vi "Create Channel.vi"(6 "units":string, 7 "index":i32, 8 "error in":errorcluster, 9 "type":T1, 10 "name":string, 11 "channel in":refnum<class "Channel.lvclass">) -> (0 "error out":errorcluster, 3 "channel out":refnum<class "Channel.lvclass">)   [LabVIEW 2020, in "Scan Engine Scripting.lvlib" / "Channel.lvclass"]
uses:
  Channel.lvclass
  Type.ctl
  Channel.lvclass/Channel.ctl
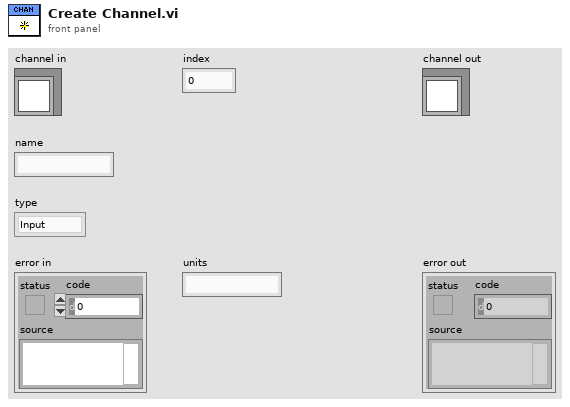
[diagram p1: front panel]
types:
  T1 = typedef "Scan Engine Scripting.lvlib/Channel.lvclass/Type.ctl" = enum16{"Input", "Output"}
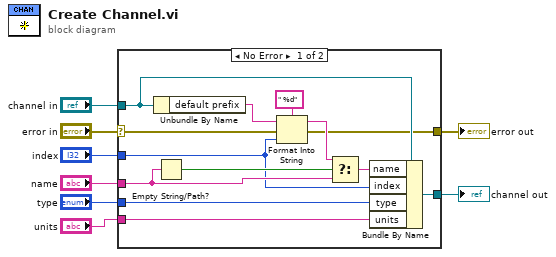
[diagram p0: block diagram]
diagram:
  n1 = case shown="No Error" "error in" {
    selector: "error in" -> [w13 w23]
    tunnel: [w12 w23] -> w7
    tunnel: [w21 w22] -> w6
    tunnel: "channel in" -> [w20 w22]
    tunnel: "name" -> [w18 _]
    tunnel: "type" -> [w10 _]
    tunnel: "units" -> [w16 _]
    tunnel: "index" -> [w9 _]
    frame No Error {
      n2 = Unbundle By Name(w20) -> ("default prefix"=w15:string)
      n3 = Empty String/Path?(string/path=w18) -> (empty?=w19:bool)
      n4 = Format Into String(format string=" %d", initial string=w15, error in=w13, w9) -> (resulting string=w14:string, error out=w12:errorcluster)
      n5 = Select(t=w14, s=w19, f=w18) -> (s? t:f=w17:string)
      n6 = Bundle By Name(cluster=w20, "name"=w17, "index"=w9, "type"=w10, "units"=w16) -> (w21:refnum<class "Channel.lvclass">)
    }
    frame Error {
    }
  }
  "error out" <- w7
  "channel out" <- w6
